vi "FGV Werte Standardanalysator.vi"(0 "FID":sgl[](array[numeric]), 1 "FID Rohwerte LIN":sgl[](array[numeric]), 5 "FID Rohwerte":sgl[](array[numeric]), 7 "PMA":sgl[](array[numeric]), 9 "PMA Rohwerte":sgl[](array[numeric]), 11 "error in (no error)":errorcluster caption="Fehler (Eingang, kein Fehler)", 12 "PMA Rohwert LIN":sgl[](array[numeric]), 13 "Aktion":T1) -> (3 "FID Rohwerte LIN":sgl[](array[numeric]), 4 "FID":sgl[](array[numeric]), 6 "FID Rohwerte":sgl[](array[numeric]), 8 "PMA":sgl[](array[numeric]), 10 "PMA Rohwerte":sgl[](array[numeric]), 14 "PMA Rohwerte LIN":sgl[](array[numeric]), 15 "error out":errorcluster caption="Fehler (Ausgang)")   [LabVIEW 2020, in "ABB-EL3000.lvlib" / "Allgemeine VI.lvlib"]
uses:
  Allgemeine VI.lvlib
  Aktion FGV Werte Standardanalysator.ctl
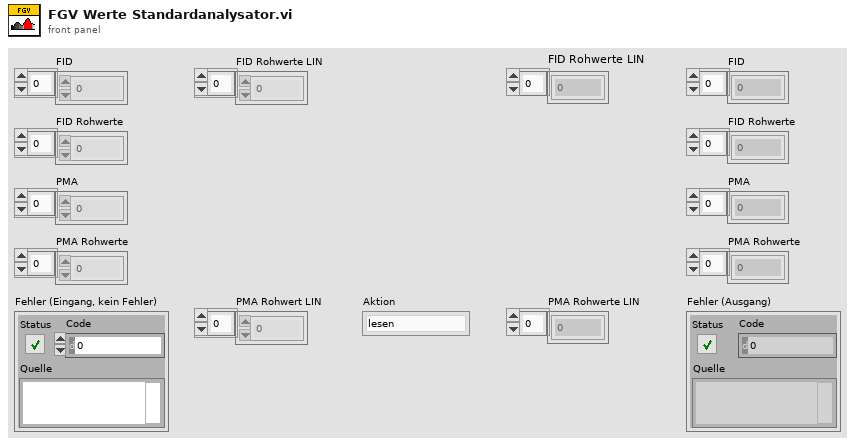
[diagram p1: front panel]
types:
  T1 = typedef "ABB-EL3000.lvlib/Allgemeine VI.lvlib/Aktion FGV Werte Standardanalysator.ctl" = enum16{"lesen", "FID", "PMA"}
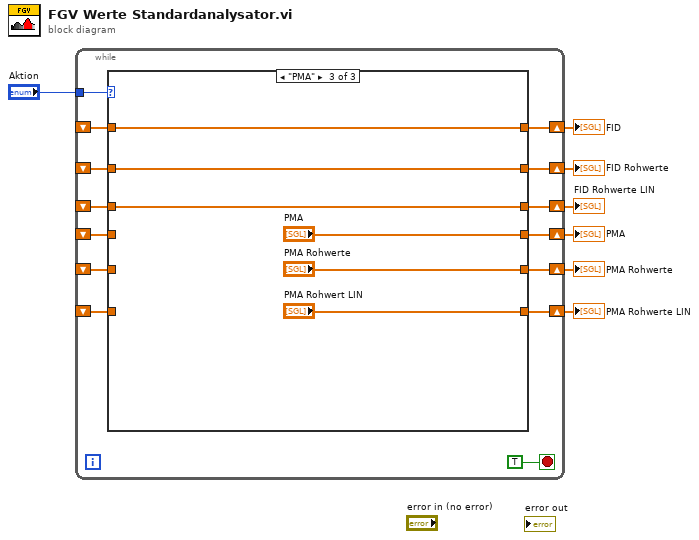
[diagram p0: block diagram]
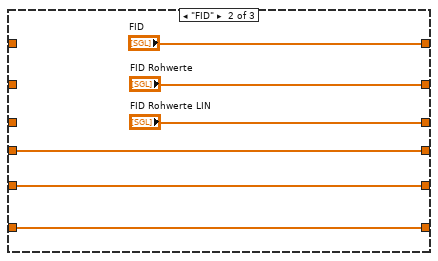
[diagram p3: hidden frame]
diagram:
  n1 = while {
    tunnel: "Aktion" -> [w20]
    shift-right: [w19] -> w6
    shift-left: _ -> [w18]
    shift-right: [w17] -> w5
    shift-left: _ -> [w16]
    shift-right: [w15] -> w4
    shift-left: _ -> [w14]
    shift-right: [w13] -> w3
    shift-left: _ -> [w12]
    shift-right: [w11] -> w2
    shift-left: _ -> [w10]
    shift-right: [w9] -> w1
    shift-left: _ -> [w8]
    stop <- TRUE stop-if-true
    n2 = case shown="\"PMA\"" w20 {
      tunnel: [w27 "FID" w39] -> w19
      tunnel: w18 -> [w27 _ w39]
      tunnel: [w26 "FID Rohwerte" w38] -> w17
      tunnel: w16 -> [w26 _ w38]
      tunnel: [w25 w31 "PMA"] -> w15
      tunnel: w14 -> [w25 w31 _]
      tunnel: [w24 w30 "PMA Rohwerte"] -> w13
      tunnel: w12 -> [w24 w30 _]
      tunnel: [w23 "FID Rohwerte LIN" w35] -> w11
      tunnel: w10 -> [w23 _ w35]
      tunnel: [w22 w28 "PMA Rohwert LIN"] -> w9
      tunnel: w8 -> [w22 w28 _]
      frame "lesen", Default {
      }
      frame "FID" {
      }
      frame "PMA" {
      }
    }
  }
  "FID" <- w6
  "FID Rohwerte" <- w5
  "PMA" <- w4
  "PMA Rohwerte" <- w3
  "FID Rohwerte LIN" <- w2
  "PMA Rohwerte LIN" <- w1
